vi "Open-TCP.vi"(8 "error in (no error)":errorcluster, 11 "SM1000-control in":T1) -> (0 "error out":errorcluster, 1 "Succes?":bool, 3 "SM1000-control out":T1)   [LabVIEW 2013, in "SLMControl.lvlib" / "SM1000.lvclass"]
uses:
  SM1000.lvclass
  Object-reference.ctl
  SM1000.lvclass/SM1000.ctl
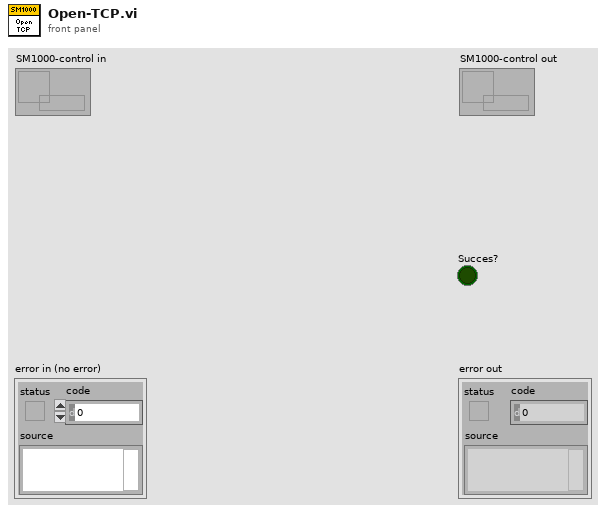
[diagram p1: front panel]
types:
  T1 = typedef "SLMControl.lvlib/SM1000.lvclass/Object-reference.ctl" = refnum<data-value>
  T2 = enum16{"Standard", "Buffered", "CRLF", "Immediate"}
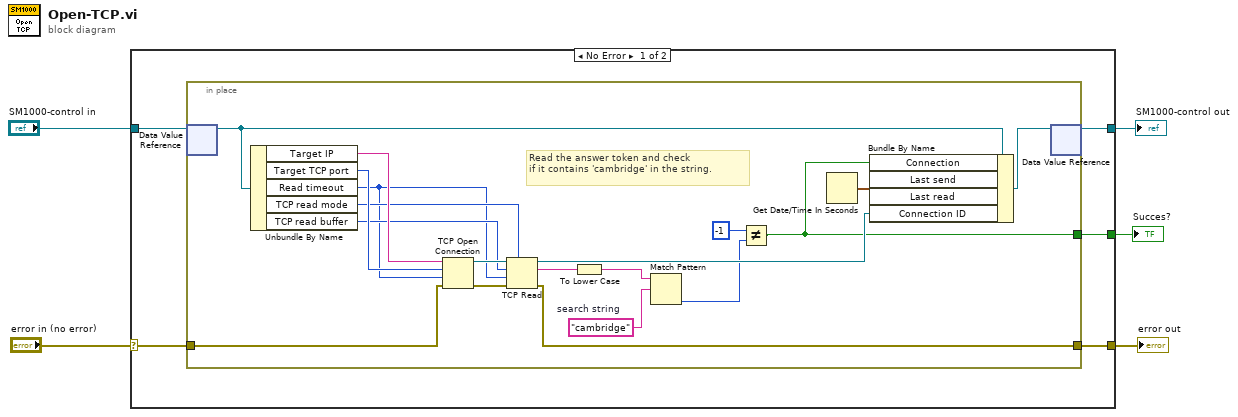
[diagram p0: block diagram]
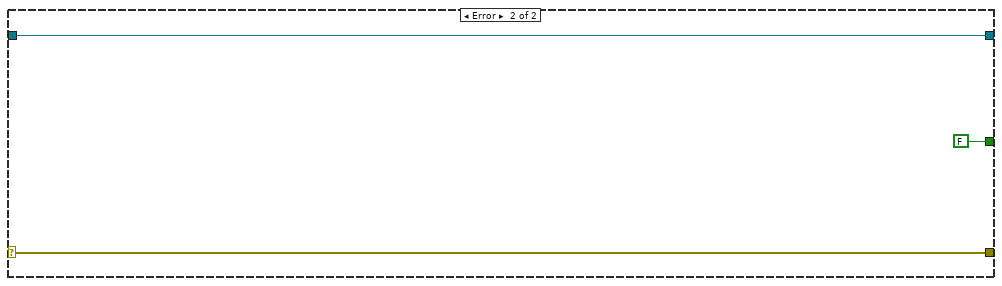
[diagram p2: hidden frame]
diagram:
  n1 = case shown="No Error" "error in (no error)" {
    selector: "error in (no error)" -> [w8 w32]
    tunnel: [w7 w32] -> w4
    tunnel: [w9 w31] -> w2
    tunnel: "SM1000-control in" -> [w10 w31]
    tunnel: [w6 FALSE] -> w1
    frame No Error {
      n2 = in-place {
        in-place-border: w8 -> [w29]
        in-place-border: [w14] -> w7
        in-place-border: [w13] -> w6
        w15 = "cambridge"  # search string
        # "Read the answer token and check \nif it contains 'cambridge' in the string."
        n3 = in-place-dvr #1(w10) -> (w26:refnum<class "SM1000.lvclass">)  [unwired: 1 out]
        n4 = Unbundle By Name(w26) -> ("Target IP"=w28:string, "Target TCP port"=w27:u16, "Read timeout"=w18:i32, "TCP read mode"=w20:T2, "TCP read buffer"=w19:i32)
        n5 = TCP Open Connection(address=w28, remote port or service name=w27, timeout ms (60000)=w18, error in (no error)=w29) -> (connection ID=w23:refnum<k5>, error out=w22:errorcluster)  [unwired: 1 in]
        n6 = TCP Read(connection ID=w23, bytes to read=w19, error in (no error)=w22, 7:w20, 9:w18) -> (connection ID out=w21:refnum<k5>, data out=w17:string, error out=w14:errorcluster)
        n7 = To Lower Case(string=w17) -> (all lower case string=w16:string)
        n8 = Match Pattern(string=w16, regular expression=w15) -> (offset past match=w12:i32)  [unwired: 1 in, 3 out]
        n9 = Not Equal?(x=-1, y=w12) -> (x != y?=w13:bool)
        n10 = Get Date/Time In Seconds() -> (seconds since 1Jan1904=w25:timestamp)
        n11 = Bundle By Name(cluster=w26, "Connection"=w13, "Last send"=w25, "Last read"=w25, "Connection ID"=w21) -> (w24:refnum<class "SM1000.lvclass">)
        n12 = in-place-dvr #1(w24) -> (w9:T1)  [unwired: 1 out]
      }
    }
    frame Error {
    }
  }
  "error out" <- w4
  "SM1000-control out" <- w2
  "Succes?" <- w1
